vi "RPC Method SignalStreamer_GetDataStream.vi"(8 "error in (no error)":errorcluster, 11 "OOP Server in":refnum<class "Streamer_server.lvclass">) -> (0 "error out":errorcluster, 3 "OOP Server out":refnum<class "Streamer_server.lvclass">)   [LabVIEW 2019, in "Streamer_server.lvlib" / "Streamer_server.lvclass"]
uses:
  Streamer_server.lvclass
  Streamer_server.lvclass/Streamer_server.ctl
  Signal Provider/Streamer.vi
  Signal Provider/Signal Provider.lvclass
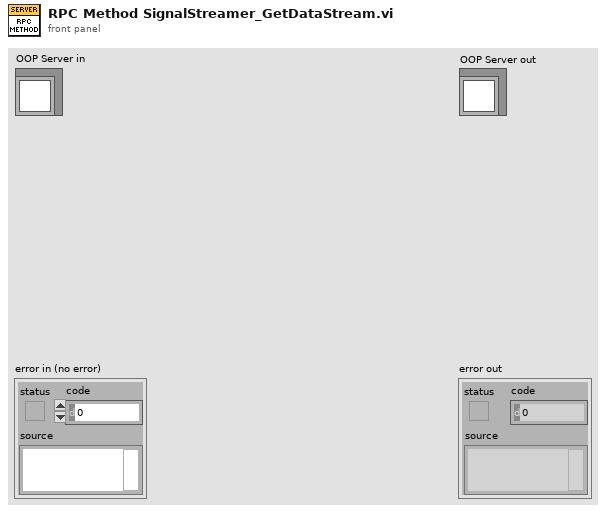
[diagram p1: front panel]
types:
  T1 = typedef "Streamer_server.lvlib/Streamer_server.lvclass/Server Internal UEs.ctl" = cluster{"SignalStreamer_GetDataStream Internal UE":refnum<user-event>}
  T2 = typedef "Streamer_server.lvlib/Streamer_server.lvclass/Server gRPC UEs.ctl" = cluster{"SignalStreamer_GetDataStream gRPC UE":refnum<user-event>}
  T3 = typedef "gprc-lvsupport-release.lvlib/grpcId.ctl" = u64
  T4 = typedef "Streamer_server.lvlib/Streamer_server.lvclass/ChannelNumber_Data.ctl" = cluster{"channel":i32}
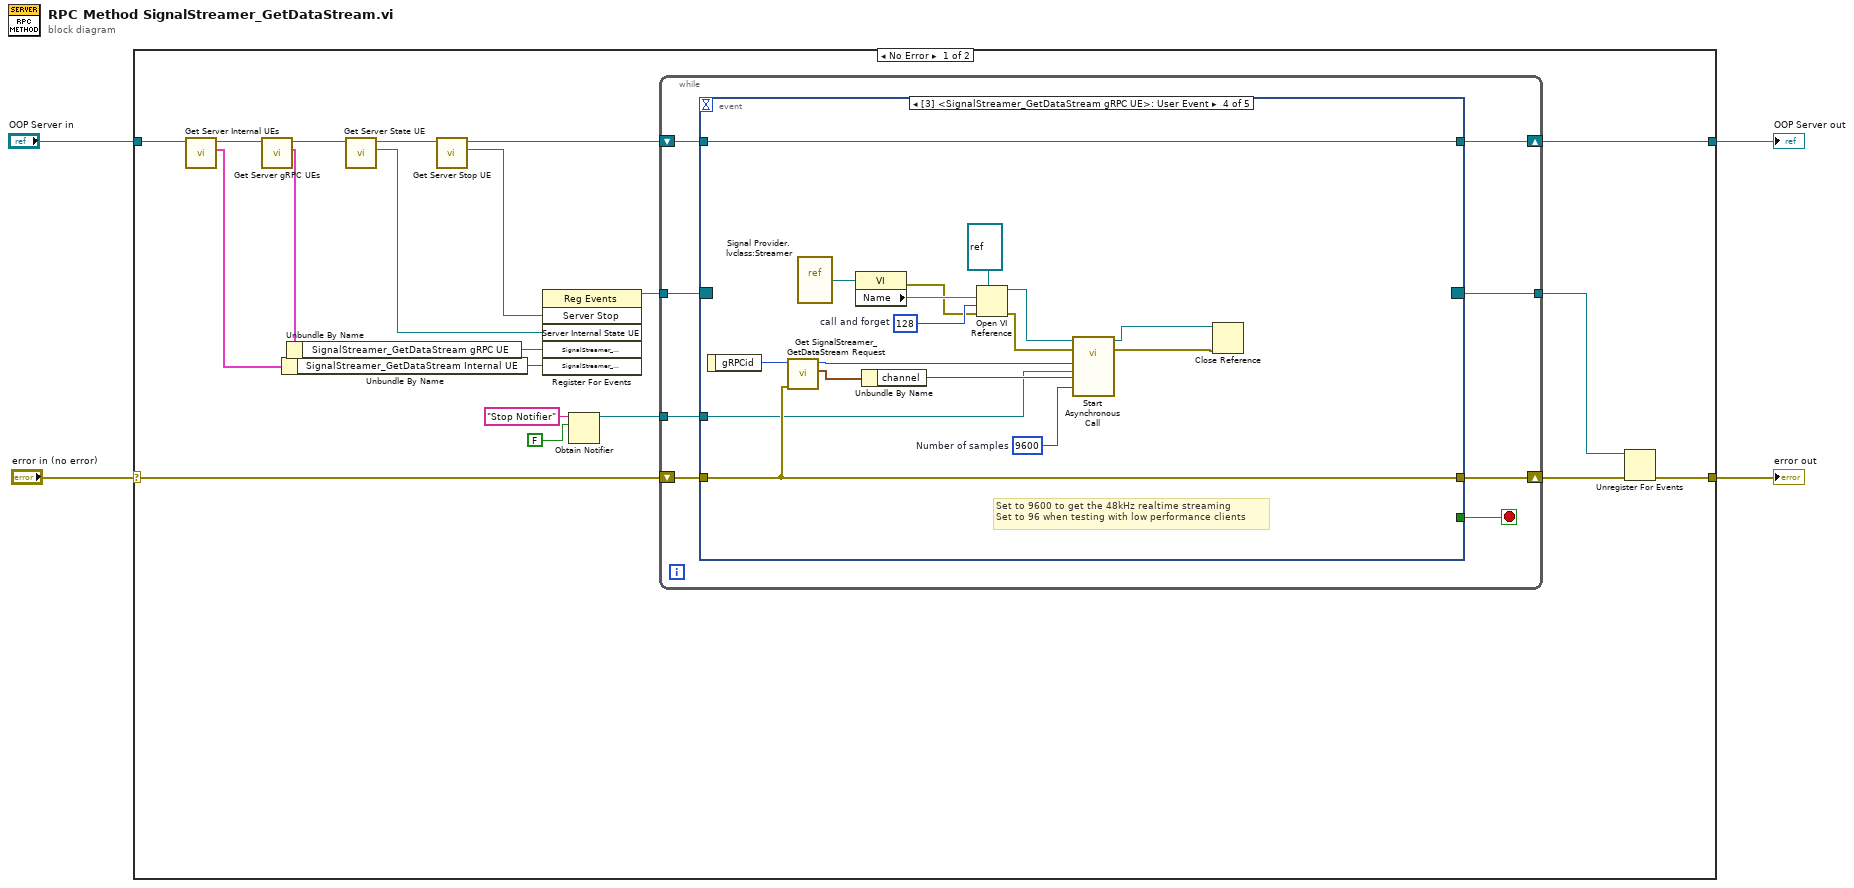
[diagram p0: block diagram]
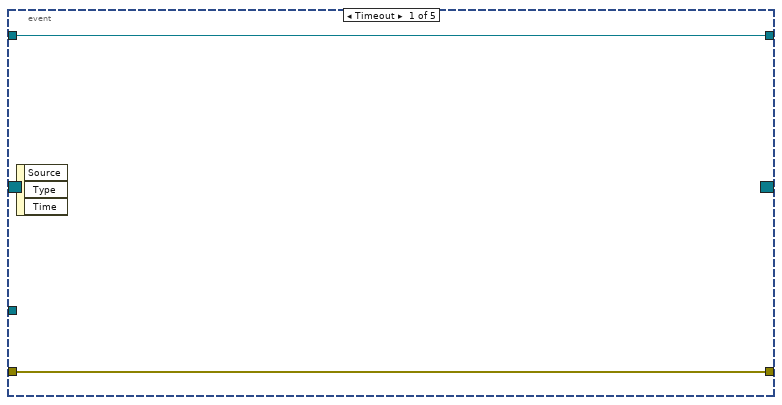
[diagram p2: hidden frame]
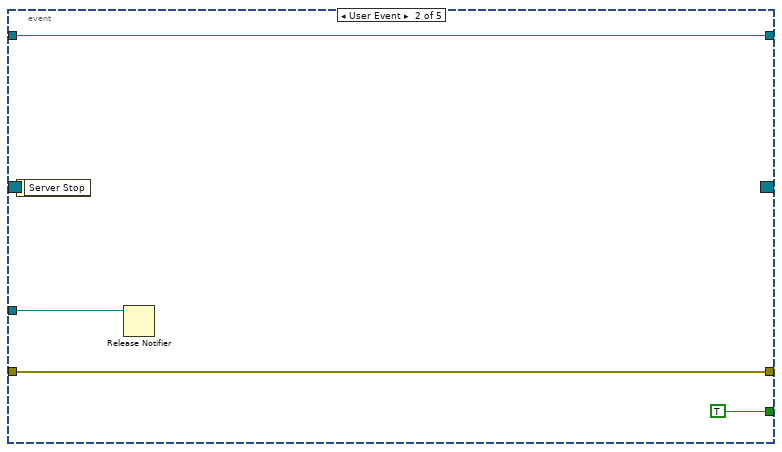
[diagram p3: hidden frame]
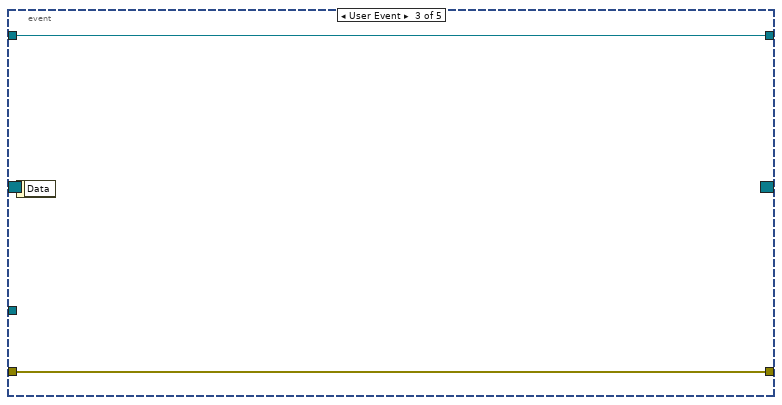
[diagram p4: hidden frame]
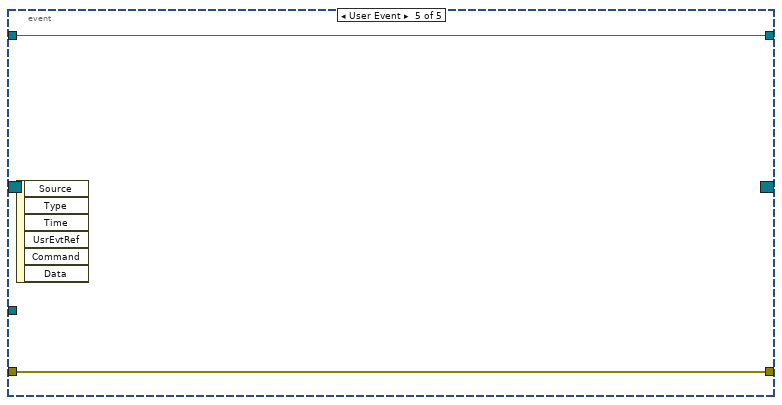
[diagram p5: hidden frame]
diagram:
  n1 = case shown="No Error" "error in (no error)" {
    selector: "error in (no error)" -> [w20 w61]
    tunnel: [w18 w61] -> w3
    tunnel: "OOP Server in" -> [w22 w60]
    tunnel: [w8 w60] -> w1
    frame No Error {
      n2 = call "Get Server Internal UEs.vi"("OOP Server in"=w22) -> ("Server Internal UEs"=w14:T1, "OOP Server out"=w21:refnum<class "Streamer_server.lvclass">)  [unwired: 9 in]
      n3 = call "Get Server gRPC UEs.vi"("OOP Server in"=w21) -> ("Server RPC Methods"=w16:T2, "OOP Server out"=w11:refnum<class "Streamer_server.lvclass">)  [unwired: 9 in]
      n4 = Unbundle By Name ("Unbundle Internal UE")(w14) -> ("SignalStreamer_GetDataStream Internal UE"=w13:refnum<user-event>)
      n5 = Unbundle By Name ("Unbundle gRPC UE")(w16) -> ("SignalStreamer_GetDataStream gRPC UE"=w15:refnum<user-event>)
      n6 = call "Get Server State UE.vi"("Template Server in"=w11) -> ("Server Internal State UE"=w9:refnum<user-event>, "Template Server out"=w10:refnum<class "Streamer_server.lvclass">)  [unwired: 9 in]
      n7 = call "Get Server Stop UE.vi"("OOP Server in"=w10) -> ("Server Stop"=w24:refnum<user-event>, "OOP Server out"=w12:refnum<class "Streamer_server.lvclass">)  [unwired: 9 in]
      n8 = register-events(w24, w9, w15, w13) -> (reference out=w23:refnum<event-registration>)  [unwired: 2 in, 1 out]
      n9 = Obtain Notifier(name (unnamed)="Stop Notifier", notification data type=FALSE) -> (notifier out=w5:refnum<notifier>)  [unwired: 2 in, 2 out]
      n10 = while {
        tunnel: w23 -> [w32]
        tunnel: [w28] -> w17
        shift-right: [w29] -> w19
        shift-left: w20 -> [w30]
        shift-right: [w26] -> w8
        shift-left: w12 -> [w27]
        tunnel: w5 -> [w25]
        stop <- w31 stop-if-true
        n11 = event "RPC Method Event Structure" shown="[3] <SignalStreamer_GetDataStream gRPC UE>: User Event" {
          selector: w32 -> [_ _ _ _ _]
          dyn-events: [_ _ _ _ _] -> w28
          timeout: _ -> [_ _ _ _ _]
          tunnel: [_ TRUE _ _ _] -> w31
          tunnel: w30 -> [w34 w37 w40 w55 w59]
          tunnel: [w34 w37 w40 w55 w59] -> w29
          tunnel: w27 -> [w33 w36 w39 w57 w58]
          tunnel: [w33 w36 w39 w57 w58] -> w26
          tunnel: w25 -> [_ w35 _ w44 _]
          event Timeout {
            n12 = event-data() -> ()  [unwired: 1 in, 3 out]
          }
          event User Event {
            n13 = event-data() -> ()  [unwired: 1 in, 1 out]
            n14 = Release Notifier(notifier=w35) -> ()  [unwired: 2 in, 3 out]
          }
          event User Event {
            n15 = event-data() -> ()  [unwired: 1 in, 1 out]
          }
          event User Event {
            w41 = 9600  # Number of samples
            w54 = 128  # call and forget
            # "Set to 9600 to get the 48kHz realtime streaming\nSet to 96 when testing with low performance clients"
            n16 = event-data() -> ("gRPCid"=w56:T3)  [unwired: 1 in]
            n17 = call "Get SignalStreamer_GetDataStream Request.vi"("error in (no error)"=w55, "gRPCid in"=w56) -> ("Message Data"=w46:T4, "gRPCid out"=w47:T3)  [unwired: 7 in, 1 out]
            n18 = vi-ref "Signal Provider.lvclass:Streamer.vi"() -> (w50:refnum<vi>)
            n19 = property class="VI"(reference=w50) -> (error out=w52:errorcluster, "Name"=w53:string)  [unwired: 1 in, 1 out]
            n20 = Unbundle By Name(w46) -> ("channel"=w45:i32)
            n21 = Open VI Reference(type specifier VI Refnum (for type only)=refnum<vi> refnum, vi path=w53, options=w54, error in (no error)=w52) -> (vi reference=w49:refnum<vi>, error out=w48:errorcluster)  [unwired: 2 in]
            n22 = call-by-ref "Start Asynchronous Call"(reference=w49, error in=w48, "#s"=w41, "channel number"=w45, "stop notifier"=w44, "gRPCid in"=w47) -> (reference out=w43:refnum<vi>, error out=w42:errorcluster)  [unwired: 8 in]
            n23 = Close Reference(reference=w43, error in (no error)=w42) -> ()  [unwired: 1 out]
          }
          event User Event {
            n24 = event-data() -> ()  [unwired: 1 in, 6 out]
          }
        }
      }
      n25 = Unregister For Events(event registration refnum=w17, error in=w19) -> (error out=w18:errorcluster)
    }
    frame Error {
    }
  }
  "error out" <- w3
  "OOP Server out" <- w1
